vi "Setup.vi"(8 "error in (no error)":errorcluster, 11 "Dummy In":refnum<class "Dummy.lvclass">) -> (0 "error out":errorcluster, 3 "Dummy Out":refnum<class "Dummy.lvclass">)   [LabVIEW 2020, in "Dummy.lvclass"]
doc: "Setup"
uses:
  Dummy.lvclass
  Dummy.lvclass/Dummy.ctl
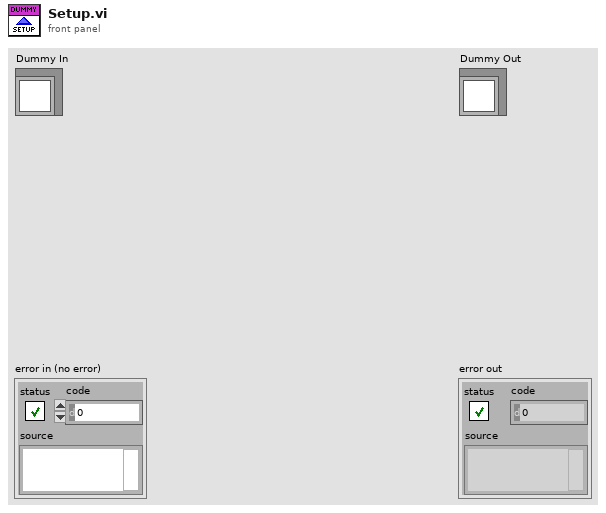
[diagram p1: front panel]
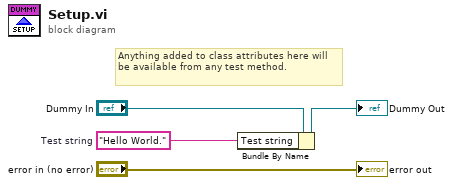
[diagram p0: block diagram]
diagram:
  w1 = "Hello World."  # Test string
  # "Anything added to class attributes here will be available from any test method."
  n1 = Bundle By Name(cluster="Dummy In", "Test string"=w1) -> (→"Dummy Out":refnum<class "Dummy.lvclass">)
  "error out" <- "error in (no error)"
